vi "AMZ_S3_APIHLP_Multipart Upload Data FG VI Ref Type.vi"() -> (0 "VI Refnum (Multipart Upload Data FG.vi Type)":refnum<vi>)   [LabVIEW 2015, in "LV Interface for Amazon S3.lvlib"]
uses:
  LV Interface for Amazon S3.lvlib
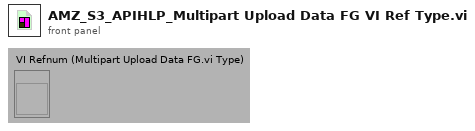
[diagram p1: front panel]
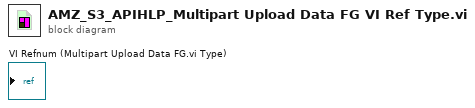
[diagram p0: block diagram]
diagram:
